vi "HP81110A Query Display.vi"(8 "error in (no error)":errorcluster, 11 "VISA session":refnum<visa-resource-name>) -> (0 "error out":errorcluster, 2 "Display (F:Off)":bool, 3 "dup VISA session":refnum<visa-resource-name>)   [LabVIEW 2009]
doc: "This VI turns the frontpanel display on and off. Switching off the display improves the programming speed of the instrument."
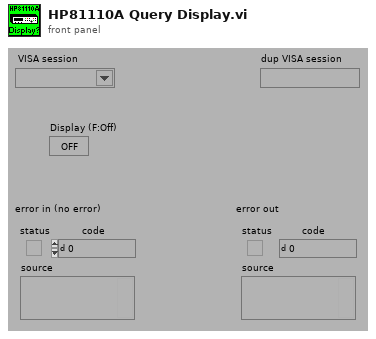
[diagram p1: front panel]
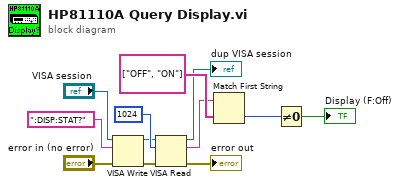
[diagram p0: block diagram]
diagram:
  n1 = VISA Write(VISA resource name="VISA session", write buffer=":DISP:STAT?", error in (no error)="error in (no error)") -> (VISA resource name out=w5:refnum<visa-resource-name>, error out=w6:errorcluster)  [unwired: 1 out]
  n2 = VISA Read(VISA resource name=w5, byte count=u32 1024 ("byte count (0)"), error in (no error)=w6) -> (VISA resource name out=→"dup VISA session":refnum<visa-resource-name>, read buffer=w8:string, error out=→"error out":errorcluster)  [unwired: 1 out]
  n3 = Match First String(2:string[] ["OFF", "ON"] ("string array"), 3:w8) -> (0:w7:i32)  [unwired: 1 out]
  n4 = Not Equal To 0?(x=w7) -> (x != 0?=→"Display (F:Off)":bool)
